vi "F05 Config Function Waveform.vi"(0 "MyIndex":u8, 2 "Waveform Mode":T1(ring), 5 "error in (no error)":errorcluster) -> (6 "Pass/Fail":bool, 8 "error out":errorcluster)   [LabVIEW 2015]
uses:
  <vilib>/Instr/_visa.llb/VISA Configure Serial Port (Instr).vi
panel:
  out "VISA":refnum<visa-resource-name> caption="VISA资源名称输出"
  out "resulting string":string
  # "Config the Function Waveform"
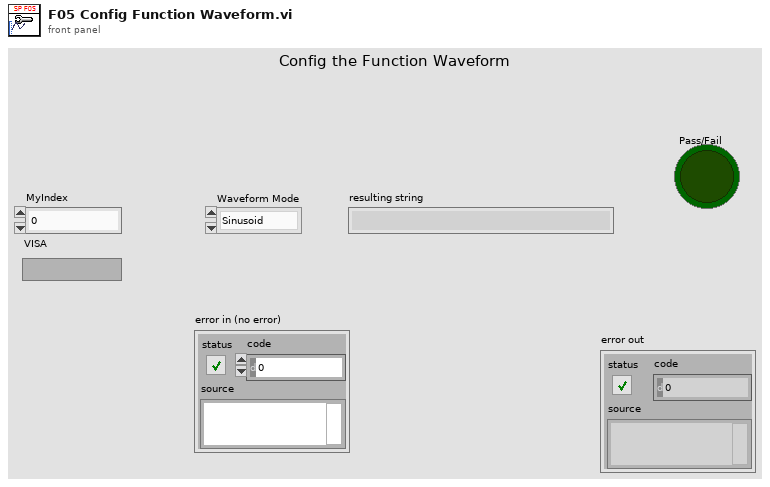
[diagram p1: front panel]
types:
  T1 = enum16{"Sinusoid", "Square", "Triangle", "UP_RAMP", "DOWN_RAMP", "Noise", "Pulse", "P_Pulse", "N_Pulse", "P_DC", "N_DC", "Query"}
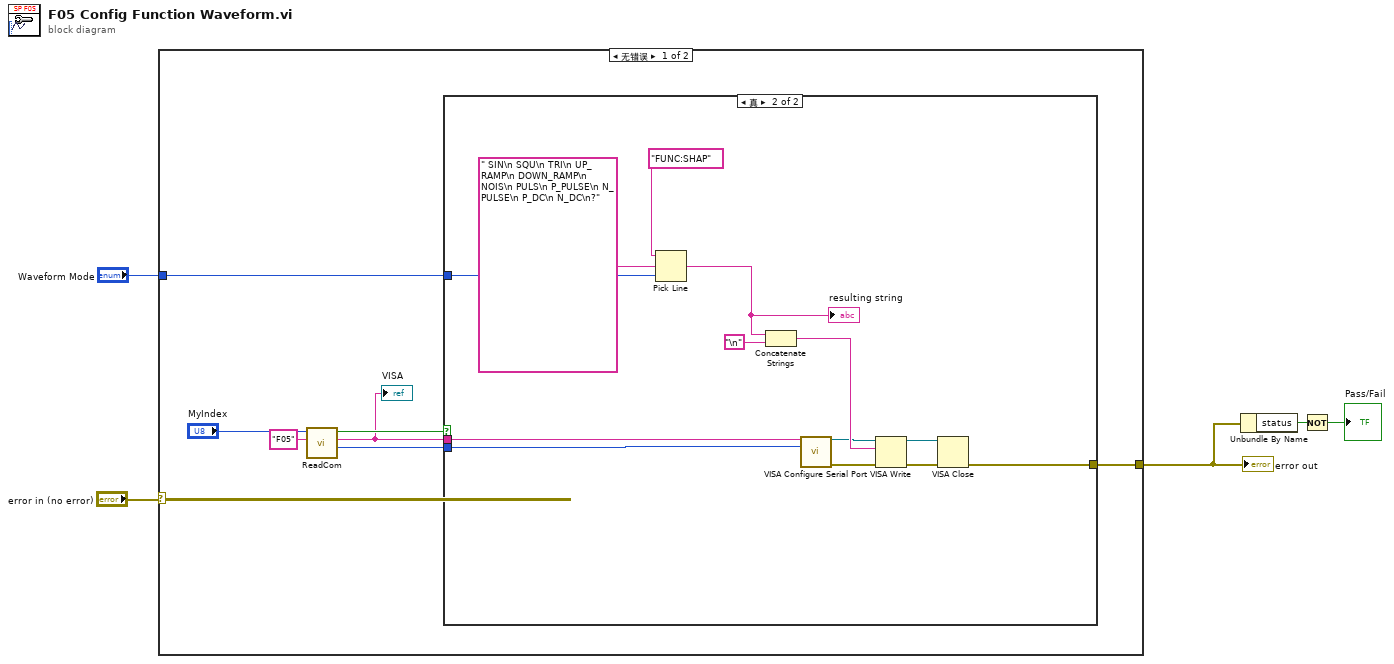
[diagram p0: block diagram]
diagram:
  n1 = case shown="无错误" "error in (no error)" {
    selector: "error in (no error)" -> [_ w26]
    tunnel: [w11 w26] -> w1
    tunnel: "Waveform Mode" -> [w12 _]
    frame No Error {
      n2 = call "ReadCom.vi"("仪器名称"="F05", "MyIndex"="MyIndex") -> ("Baudrate"=w6:i32, "COM"=w7:string, "OK?"=w8:bool)  [unwired: 7 in]
      "VISA" <- w7
      n3 = case shown="真" w8 {
        tunnel: w12 -> [_ w25]
        tunnel: [_ w17] -> w11
        tunnel: w7 -> [_ w14]
        tunnel: w6 -> [_ w13]
        frame False {
        }
        frame True {
          n4 = Pick Line(string ("")="FUNC:SHAP" ("字符串(\"\")"), multi-line string=" SIN\n SQU\n TRI\n UP_RAMP\n DOWN_RAMP\n NOIS\n PULS\n P_PULSE\n N_PULSE\n P_DC\n N_DC\n?", line index=w25) -> (output string=w20:string)
          "resulting string" <- w20
          n5 = Concatenate Strings(w20, "\n") -> (w22:string)
          n6 = call-poly "VISA Configure Serial Port"("VISA resource name"=w14, "baud rate (9600)"=w13) -> ("VISA resource name out"=w16:refnum<visa-resource-name>, "error out"=w15:errorcluster)  [unwired: 12 in]
          n7 = VISA Write(VISA resource name=w16, write buffer=w22, error in (no error)=w15) -> (VISA resource name out=w19:refnum<visa-resource-name>, error out=w18:errorcluster)  [unwired: 1 out]
          n8 = VISA Close(VISA resource name=w19, error in (no error)=w18) -> (error out=w17:errorcluster)
        }
      }
    }
    frame Error {
    }
  }
  "error out" <- w1
  n9 = Unbundle By Name(w1) -> ("status"=w2:bool)
  n10 = Not(x=w2) -> (.not. x?=→"Pass/Fail":bool)
